vi "DM get tx (mulit).vi"(8 "error in (no error)":errorcluster, 11 "tx bursts":string[](array[string])) -> (0 "error out":errorcluster, 3 "1D Array":refnum<class "mmWave data.lvclass">[](array[class]))   [LabVIEW 2019, in "DataManagment.lvlib"]
uses:
  DataManagment.lvlib
  SubVIs/mmWave data_class/mmWave data.lvclass
  DM get burst parameters.ctl
  c7c6d1de-ea7e-4b56-9f74-e400fa680664.vi
  <vilib>/Utility/error.llb/Error Cluster From Error Code.vi
  <vilib>/ErrorRing/Error Ring.xnode
  <vilib>/addons/_JKI.lib/Serialization/JSON/JKI JSON Serialization.lvlib
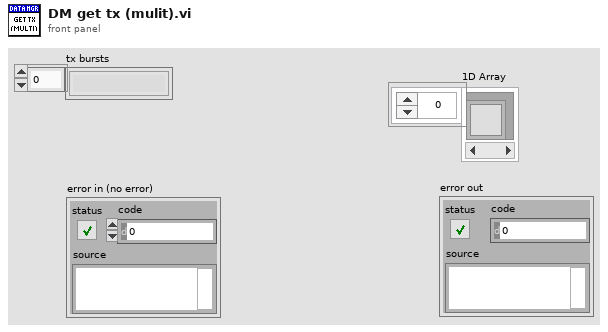
[diagram p1: front panel]
types:
  T1 = typedef "DataManagment.lvlib/DM get burst parameters.ctl" = cluster{"group":string, "bursts":string[]}
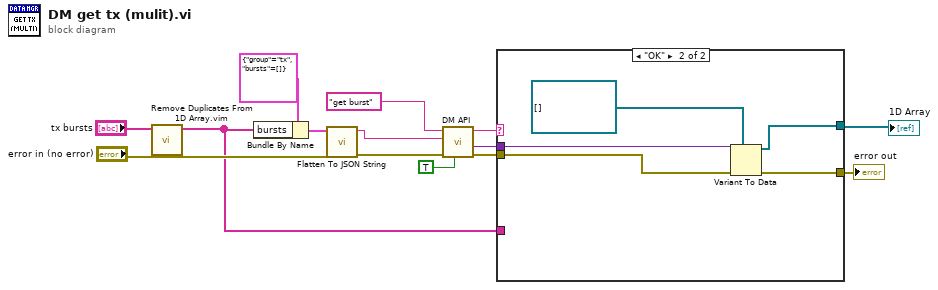
[diagram p0: block diagram]
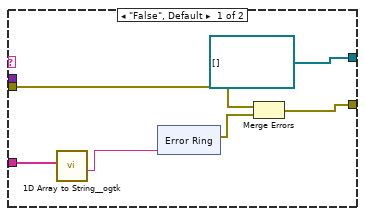
[diagram p2: hidden frame]
diagram:
  n1 = call "Remove Duplicates From 1D Array.vim"("array"="tx bursts") -> ("array with duplicates removed"=w1:string[])  [unwired: 10 in]
  n2 = Bundle By Name(cluster=T1 {"group"="tx", "bursts"=[]} ("Cluster"), "bursts"=w1) -> (w7:T1)
  n3 = call <vilib>:"Flatten To JSON String.vi"("error in (no error)"="error in (no error)", "Variant"=w7) -> ("error out"=w3:errorcluster, "JSON String"=w5:string)  [unwired: 8 in]
  n4 = call "DM API.vi"("response"=TRUE, "error in (no error)"=w3, "parameters"=w5, "message"="get burst") -> ("error out"=w11:errorcluster, "data"=w12:variant, "status"=w13:string)  [unwired: 4 in, 1 out]
  n5 = case shown="\"OK\"" w13 {
    tunnel: w12 -> [_ w32]
    tunnel: [refnum<class "mmWave data.lvclass">[] [] ("Array") w28] -> w9
    tunnel: [w18 w29] -> w10
    tunnel: w11 -> [w17 w30]
    tunnel: w1 -> [w16 _]
    frame "False", Default {
      n6 = call <userlib>:"1D Array to String__ogtk.vi"("Array of Strings"=w16) -> ("delimited string"=w15:string)  [unwired: 10 in]
      n7 = xnode "Error Ring"("parameter 0"=w15) -> ("error out"=w19:errorcluster)
      n8 = Merge Errors(w17, w19) -> (w18:errorcluster)
    }
    frame "OK" {
      n9 = Variant To Data(error in=w30, type=refnum<class "mmWave data.lvclass">[] [] ("Array"), Variant=w32) -> (data=w28:refnum<class "mmWave data.lvclass">[], error out=w29:errorcluster)
    }
  }
  "error out" <- w10
  "1D Array" <- w9
